vi "Angle Corrections.vi"(11 "Image array":dbl[][](array[numeric])) -> (3 "Image array_Cos_Correction":dbl[][](array[numeric]))   [LabVIEW 2018]
uses:
  Global Variables.vi
  <vilib>/imath/engines/lvmath2/RunTimeEngine/BuiltInFunctions/atan/NIMS_atan(C).vi
  <instcachedir>/0/NIMS_atan(C)_D8A4E8999A304D6BADBC2037B8EF9094.lvgen/NIMS_atan(C)_D8A4E8999A304D6BADBC2037B8EF9094_001.vi
  <vilib>/imath/engines/lvmath2/RunTimeEngine/BuiltInFunctions/cos/NIMS_cos(C).vi
  <instcachedir>/0/NIMS_cos(C)_BAE2C1A787AA4ECB8E8ACD00F28F4DBC.lvgen/NIMS_cos(C)_BAE2C1A787AA4ECB8E8ACD00F28F4DBC_001.vi
  <vilib>/imath/engines/lvmath2/RunTimeEngine/NodeEndStatement/NIMS_NodeEndStatement_Output.vi
  <instcachedir>/0/NIMS_NodeEndStatement_Output_53EC0D466D134D7ABD903AC30B43404B.lvgen/NIMS_NodeEndStatement_Output_53EC0D466D134D7ABD903AC30B43404B_008.vi
  <vilib>/imath/engines/lvmath2/RunTimeEngine/ErrorHandling/NIMS_Finalize Error.vi
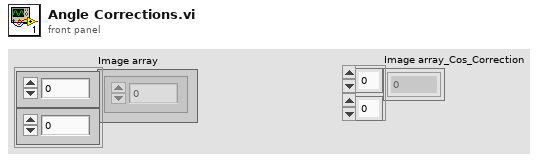
[diagram p1: front panel]
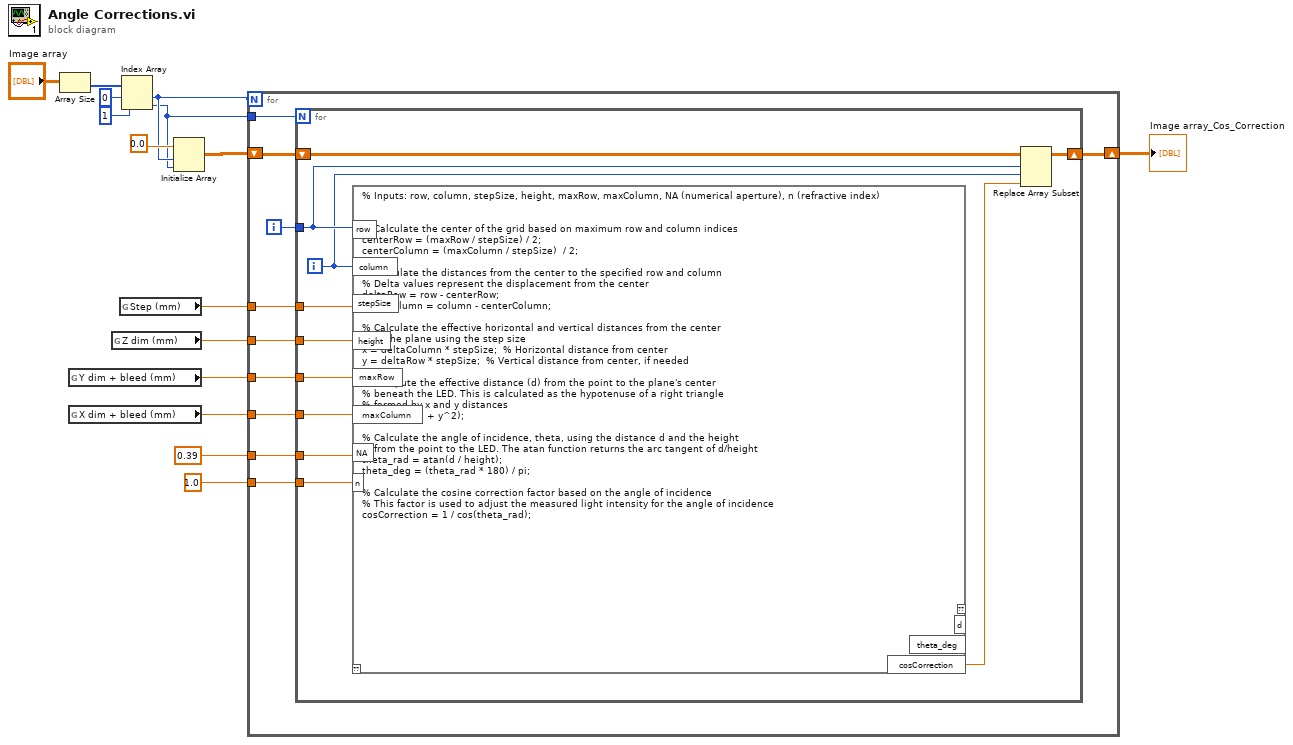
[diagram p0: block diagram]
diagram:
  n1 = Array Size(array="Image array") -> (size(s)=w15:i32[])
  n2 = global read "Global Variables.vi" "Y dim + bleed (mm)"() -> (w4:dbl)
  n3 = global read "Global Variables.vi" "X dim + bleed (mm)"() -> (w3:dbl)
  n4 = global read "Global Variables.vi" "Z dim (mm)"() -> (w5:dbl)
  n5 = global read "Global Variables.vi" "Step (mm)"() -> (w6:dbl)
  n6 = Index Array(array=w15, index #1=0 ("index"), index #2=1 ("index")) -> (element #1=w2:i32, element #2=w1:i32)
  n7 = Initialize Array(0.0, w2, w1) -> (w7:dbl[][])
  n8 = for {
    N: w2 -> [_]
    shift-right: [w23] -> w9
    shift-left: w7 -> [w24]
    tunnel: 0.39 ("NA") -> [w22]
    tunnel: 1.0 ("n") -> [w21]
    tunnel: w6 -> [w20]
    tunnel: w5 -> [w19]
    tunnel: w4 -> [w18]
    tunnel: w3 -> [w17]
    tunnel: w1 -> [w16]
    i -> [w25]
    n9 = for {
      N: w16 -> [_]
      tunnel: w25 -> [w32]
      shift-right: [w35] -> w23
      shift-left: w24 -> [w36]
      tunnel: w22 -> [w34]
      tunnel: w21 -> [w33]
      tunnel: w20 -> [w29]
      tunnel: w19 -> [w28]
      tunnel: w18 -> [w27]
      tunnel: w17 -> [w26]
      i -> [w31]
      n10 = mathscript code="% Inputs: row, column, stepSize, height, maxRow, maxColumn, NA (numerical aperture), n (refractive index)\n\n\n% Calculate the center of the grid based on maximum row and column indices\ncenterRow = (maxRow / stepSize) / 2;\ncenterColumn = (maxColumn / stepSize)  / 2;\n\n% Calculate the distances from the center to the specified row and column\n% Delta values represent the displacement from the center\ndeltaRow = row - centerRow;\ndeltaColumn = column - centerColumn;\n\n% Calculate the effective horizontal and vertical distances from the center\n% of the plane using the step size\nx = deltaColumn * stepSize;  % Horizontal distance from center\ny = deltaRow * stepSize;  % Vertical distance from center, if needed\n\n% Compute the effective distance (d) from the point to the plane's center\n% beneath the LED. This is calculated as the hypotenuse of a right triangle\n% formed by x and y distances\nd = sqrt(x^2 + y^2);\n\n% Calculate the angle of incidence, theta, using the distance d and the height\n% from the point to the LED. The atan function returns the arc tangent of d/height\ntheta_rad = atan(d / height);\ntheta_deg = (theta_rad * 180) / pi;\n\n% Calculate the cosine correction factor based on the angle of incidence\n% This factor is used to adjust the measured light intensity for the angle of incidence\ncosCorrection = 1 / cos(theta_rad);"("row"=w32, "column"=w31, "stepSize"=w29, "height"=w28, "maxRow"=w27, "maxColumn"=w26, "NA"=w34, "n"=w33) -> ("cosCorrection"=w30:cdb)  [unwired: 1 in, 3 out]
      n11 = Replace Array Subset(array=w36, new element=w30, index (row)=w32, index (col)=w31) -> (w35:dbl[][])
    }
  }
  "Image array_Cos_Correction" <- w9
